vi "LogSourceData.vi"(0 "LogFilePath":path, 1 "DECsonde":dbl format="%<%H:%M:%S>t", 2 "RAsonde":dbl format="%<%H:%M:%S%1u>t", 5 "TimeStampTreshold":dbl format="%<%H:%M:%S%1u\n%x>T", 7 "SNR IN":cluster{dbl[], dbl[]}[](array[cluster]) {"?" format="%<%H:%M:%S%1u\n%x>T"}, 9 "Flux IN":cluster{dbl[], dbl[]}[](array[cluster]) {"?" format="%<%H:%M:%S%1u>T"}, 11 "Centroids IN":cluster{dbl[], dbl[]}[](array[cluster]) {"?" format="%<%H:%M:%S%1u>T"}) -> (15 "String":string)   [LabVIEW 2019]
panel:
  out "length":i32
  out "size_ap":i32
  out "size_av":i32
  out "TresholdIndex":i32
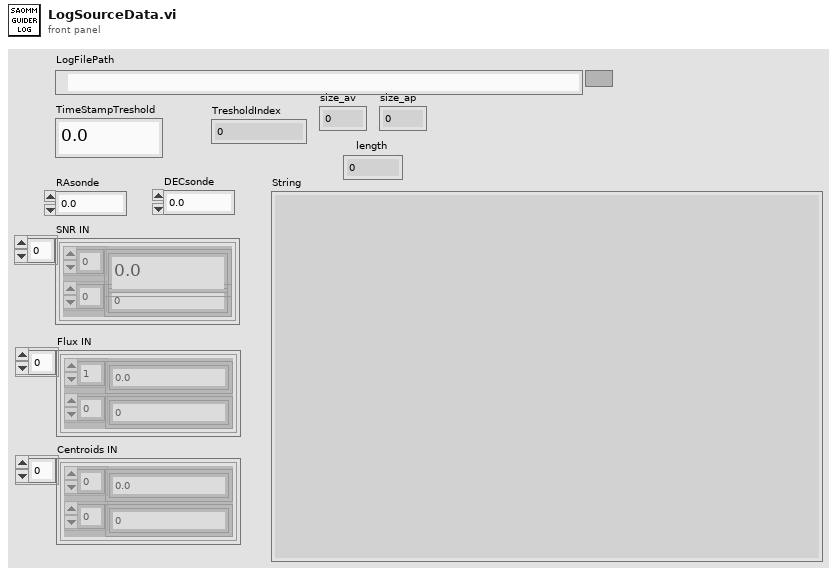
[diagram p1: front panel]
types:
  T1 = typedef "LVDateTimeRec.ctl" = cluster{"fractional second":dbl, "second":i32, "minute":i32, "hour":i32, "day of month":i32, "month":i32, "year":i32, "day of week":i32, "day of year":i32, "DST":i32}
  T2 = enum16{"open", "replace", "create", "open or create", "replace or create", "replace or create with confirmation"}
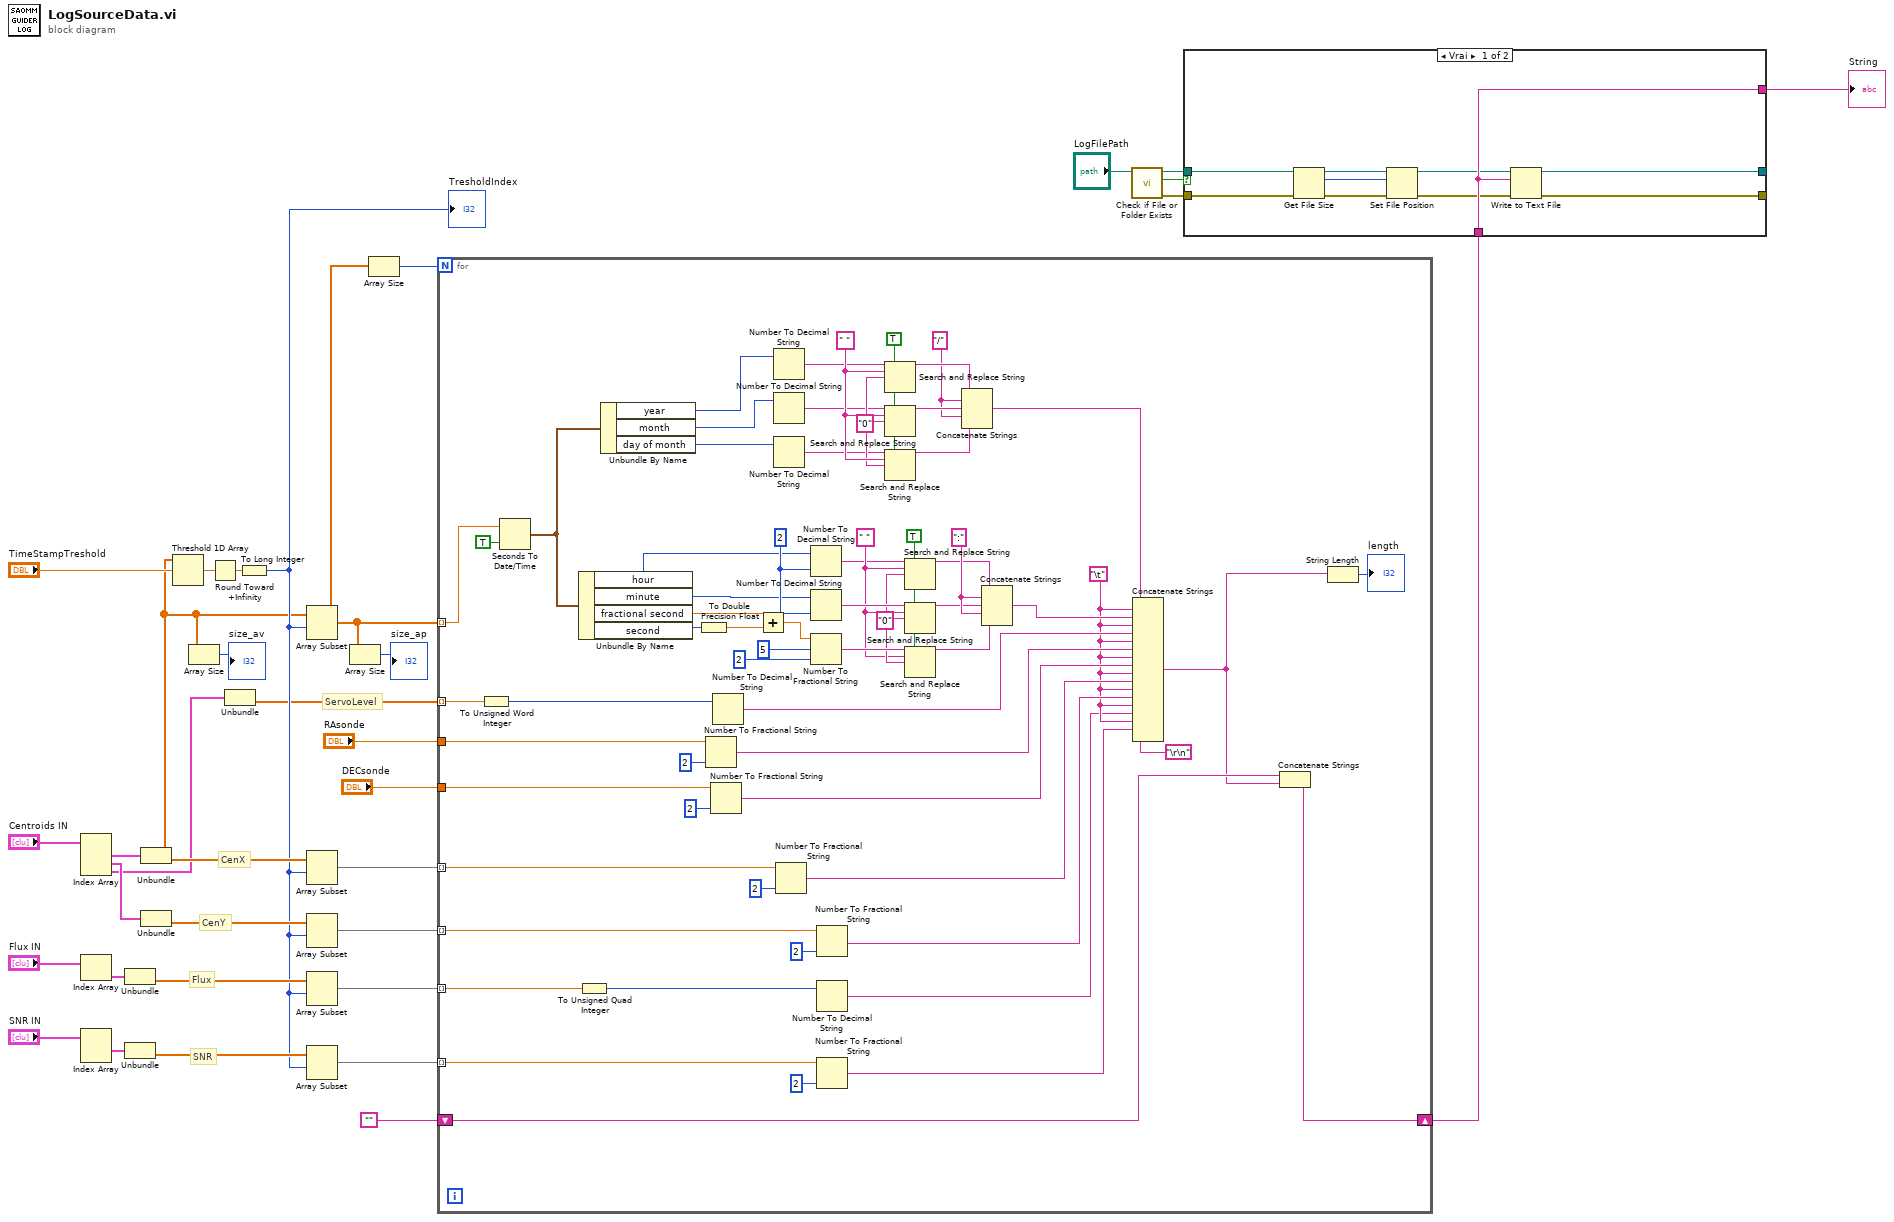
[diagram p0: block diagram]
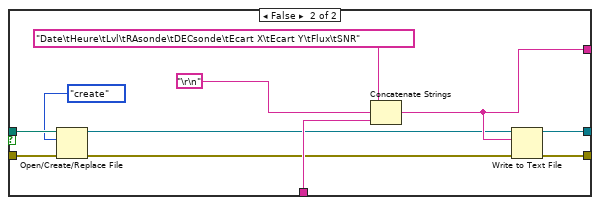
[diagram p2: hidden frame]
diagram:
  # "SNR"
  # "Flux"
  # "CenY"
  # "CenX"
  # "ServoLevel"
  n1 = Index Array(array="Centroids IN") -> (element #1=w35:cluster{dbl[], dbl[]}, element #2=w31:cluster{dbl[], dbl[]}, element #3=w2:cluster{dbl[], dbl[]})  [unwired: 3 in]
  n2 = Index Array(array="Flux IN") -> (element=w29:cluster{dbl[], dbl[]})  [unwired: 1 in]
  n3 = Index Array(array="SNR IN") -> (element #1=w28:cluster{dbl[], dbl[]})  [unwired: 2 in, 1 out]
  n4 = Unbundle(w29) -> (w27:dbl[])  [unwired: 1 out]
  n5 = Unbundle(w28) -> (w26:dbl[])  [unwired: 1 out]
  n6 = Unbundle(w35) -> (w16:dbl[], w32:dbl[])
  n7 = Unbundle(w31) -> (w30:dbl[])  [unwired: 1 out]
  n8 = Threshold 1D Array(2:"TimeStampTreshold", 3:w16) -> (0:w33:dbl)  [unwired: 1 in]
  n9 = Array Size(array=w16) -> (size(s)=→"size_av":i32)
  n10 = Round Toward +Infinity(x=w33) -> (ceil(x): smallest int >= x=w25:dbl)
  n11 = Unbundle(w2) -> (w1:dbl[])  [unwired: 1 out]
  n12 = To Long Integer(number=w25) -> (32bit integer=w24:i32)
  "TresholdIndex" <- w24
  n13 = Array Subset(array=w16, index=w24) -> (w14:dbl[])  [unwired: 1 in]
  n14 = Array Subset(array=w32, index=w24) -> (w11:dbl[])  [unwired: 1 in]
  n15 = Array Subset(array=w30, index=w24) -> (w12:dbl[])  [unwired: 1 in]
  n16 = Array Subset(array=w27, index=w24) -> (w22:dbl[])  [unwired: 1 in]
  n17 = Array Subset(array=w26, index=w24) -> (w21:dbl[])  [unwired: 1 in]
  n18 = Array Size(array=w14) -> (size(s)=→"size_ap":i32)
  n19 = Array Size(array=w14) -> (size(s)=w23:i32)
  n20 = for {
    N: w23 -> [_]
    tunnel: w14 -> [w86] mode=indexing
    tunnel: w11 -> [w80] mode=indexing
    tunnel: w12 -> [w79] mode=indexing
    tunnel: w22 -> [w78] mode=indexing
    tunnel: w21 -> [w84] mode=indexing
    shift-right: [w75] -> w6
    shift-left: "" -> [w76]
    tunnel: "RAsonde" -> [w52]
    tunnel: "DECsonde" -> [w51]
    tunnel: w1 -> [w50] mode=indexing
    w64 = "/"
    w59 = TRUE ("replace all? (F)")
    w68 = "0" ("replace string (\"\")")
    w69 = " " ("search string")
    w43 = "\t"
    w99 = ":"
    w60 = TRUE ("replace all? (F)")
    w93 = "0" ("replace string (\"\")")
    w92 = " " ("search string")
    w90 = i16 2 ("width (-)")
    n21 = To Unsigned Word Integer(number=w50) -> (unsigned 16bit integer=w49:u16)
    n22 = Seconds To Date/Time(time stamp (now)=w86, to UTC (F)=TRUE) -> (date time rec=w70:T1)
    n23 = Unbundle By Name(w70) -> ("hour"=w89:i32, "minute"=w88:i32, "fractional second"=w38:dbl, "second"=w37:i32)
    n24 = To Unsigned Quad Integer(1:w78) -> (0:w77:u64)
    n25 = Unbundle By Name(w70) -> ("year"=w58:i32, "month"=w57:i32, "day of month"=w56:i32)
    n26 = To Double Precision Float(number=w37) -> (double precision float=w39:dbl)
    n27 = Number To Fractional String(number=w52, precision (6)=i16 2) -> (F-format string=w47:string)  [unwired: 2 in]
    n28 = Number To Fractional String(number=w51, precision (6)=i16 2) -> (F-format string=w46:string)  [unwired: 2 in]
    n29 = Number To Decimal String(number=w49) -> (decimal integer string=w48:string)  [unwired: 1 in]
    n30 = Add(x=w38, y=w39) -> (x+y=w36:dbl)
    n31 = Number To Decimal String(number=w58) -> (decimal integer string=w63:string)  [unwired: 1 in]
    n32 = Number To Decimal String(number=w57) -> (decimal integer string=w62:string)  [unwired: 1 in]
    n33 = Number To Decimal String(number=w56) -> (decimal integer string=w61:string)  [unwired: 1 in]
    n34 = Number To Fractional String(number=w80, precision (6)=i16 2) -> (F-format string=w45:string)  [unwired: 2 in]
    n35 = Number To Decimal String(number=w89, width (-)=w90) -> (decimal integer string=w91:string)
    n36 = Number To Decimal String(number=w88, width (-)=w90) -> (decimal integer string=w94:string)
    n37 = Number To Fractional String(number=w36, width (-)=i16 5, precision (6)=i16 2) -> (F-format string=w95:string)  [unwired: 1 in]
    n38 = Number To Fractional String(number=w79, precision (6)=i16 2) -> (F-format string=w44:string)  [unwired: 2 in]
    n39 = Number To Decimal String(number=w77) -> (decimal integer string=w41:string)  [unwired: 1 in]
    n40 = Number To Fractional String(number=w84, precision (6)=i16 2) -> (F-format string=w40:string)  [unwired: 2 in]
    n41 = Search and Replace String(replace all?=w59, input string=w63, search string=w69, replace string=w68) -> (result string=w66:string)  [unwired: 4 in, 3 out]
    n42 = Search and Replace String(replace all?=w59, input string=w62, search string=w69, replace string=w68) -> (result string=w67:string)  [unwired: 4 in, 3 out]
    n43 = Search and Replace String(replace all?=w59, input string=w61, search string=w69, replace string=w68) -> (result string=w65:string)  [unwired: 4 in, 3 out]
    n44 = Search and Replace String(replace all?=w60, input string=w91, search string=w92, replace string=w93) -> (result string=w97:string)  [unwired: 4 in, 3 out]
    n45 = Search and Replace String(replace all?=w60, input string=w94, search string=w92, replace string=w93) -> (result string=w96:string)  [unwired: 4 in, 3 out]
    n46 = Search and Replace String(replace all?=w60, input string=w95, search string=w92, replace string=w93) -> (result string=w98:string)  [unwired: 4 in, 3 out]
    n47 = Concatenate Strings(w66, w64, w67, w64, w65) -> (w55:string)
    n48 = Concatenate Strings(w97, w99, w96, w99, w98) -> (w85:string)
    n49 = Concatenate Strings(w55, w43, w85, w43, w48, w43, w47, w43, w46, w43, w45, w43, w44, w43, w41, w43, w40, "\r\n") -> (w73:string)
    n50 = Concatenate Strings(w76, w73) -> (w75:string)
    n51 = String Length(string=w73) -> (length=→"length":i32)
  }
  n52 = call <vilib>:"Check if File or Folder Exists.vi"("path"="LogFilePath") -> ("error out"=w7:errorcluster, "file or folder exists?"=w9:bool, "dup path"=w8:path)  [unwired: 8 in]
  n53 = case shown="Vrai" w9 {
    tunnel: w8 -> [w103 w120]
    tunnel: w7 -> [w102 w119]
    tunnel: [w109 w118] -> _
    tunnel: [w108 w117] -> _
    tunnel: w6 -> [w107 w116]
    tunnel: [w107 w115] -> w5
    frame True {
      n54 = Get File Size(file=w103, error in=w102) -> (refnum out=w106:refnum<file>, size (in bytes)=w105:i64, 0:w104:errorcluster)
      n55 = Set File Position(offset (in bytes) (0)=w105, refnum=w106, error in=w104) -> (refnum out=w101:refnum<file>, error out=w100:errorcluster)  [unwired: 1 in]
      n56 = Write to Text File(file (use dialog)=w101, text=w107, error in=w100) -> (refnum out=w109:refnum<file>, error out=w108:errorcluster)  [unwired: 1 in, 1 out]
    }
    frame False {
      n57 = Open/Create/Replace File(file path (use dialog)=w120, error in=w119, operation (0:open)=T2."create") -> (refnum out=w111:refnum<file>, error out=w110:errorcluster)  [unwired: 3 in, 1 out]
      n58 = Concatenate Strings("Date\tHeure\tLvl\tRAsonde\tDECsonde\tEcart X\tEcart Y\tFlux\tSNR", "\r\n", w116) -> (w115:string)
      n59 = Write to Text File(file (use dialog)=w111, text=w115, error in=w110) -> (refnum out=w118:refnum<file>, error out=w117:errorcluster)  [unwired: 1 in, 1 out]
    }
  }
  "String" <- w5
